vi "convert_time_with_functions.vi"() -> ()   [LabVIEW 2021]
uses:
  <vilib>/Utility/miscctls.llb/LVDateTimeRec.ctl
panel:
  out "time stamp 2":timestamp
  out "time stamp":timestamp
  out "date time rec":T1
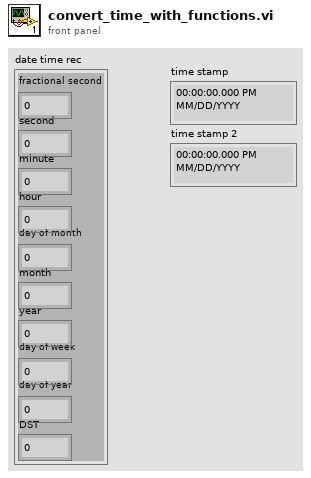
[diagram p1: front panel]
types:
  T1 = typedef "LVDateTimeRec.ctl" = cluster{"fractional second":dbl, "second":i32, "minute":i32, "hour":i32, "day of month":i32, "month":i32, "year":i32, "day of week":i32, "day of year":i32, "DST":i32}
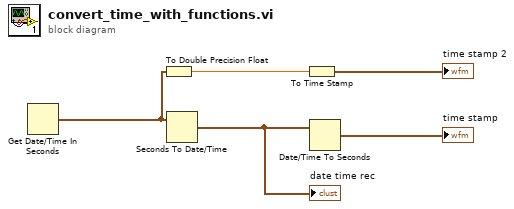
[diagram p0: block diagram]
diagram:
  n1 = Get Date/Time In Seconds() -> (seconds since 1Jan1904=w4:timestamp)
  n2 = To Double Precision Float(number=w4) -> (double precision float=w5:dbl)
  n3 = Seconds To Date/Time(time stamp (now)=w4) -> (date time rec=w1:T1)  [unwired: 1 in]
  "date time rec" <- w1
  n4 = To Time Stamp(1:w5) -> (0:→"time stamp 2":timestamp)
  n5 = Date/Time To Seconds(2:w1) -> (0:→"time stamp":timestamp)  [unwired: 1 in]
